vi "main.vi"() -> ()   [LabVIEW 2010]
uses:
  common_typedefs/channels_cluster.ctl
  common_typedefs/gate_parameters_cluster.ctl
  FPGAsubVIs/OnBoardBuffer/OnBoardBuffer.ctl
  FPGAsubVIs/write-to-fifo_status.ctl
  <vilib>/Platform/TimedLoop/XDataNode/XDataNode.xnode
  <vilib>/Platform/TimedLoop/XDataNode/timing_clust.ctl
  <vilib>/Platform/TimedLoop/XDataNode/nitl_modes.ctl
  <vilib>/Platform/TimedLoop/XDataNode/wakeup.ctl
  <vilib>/rvi/DataTransferAndStorage/Container/XNode/niFpgaContainer.xnode
  <vilib>/rvi/FIFO/Fifo_Resource/nirvififoEmulationSetSize.vi
  <vilib>/rvi/DataTransferAndStorage/Container/Common/niFpgaContainerGetUniqueNameForEmu.vi
  <vilib>/Platform/TimedLoop/XDataNode/XDNodeRunTimeDep.lvlib
  FPGAsubVIs/OnBoardBuffer/OnBoardBuffer.lvlib
panel:
  in  "clamp first pixel?":bool
  out "data received for buffering":u64
  out "local transfer FIFO full?":bool
  out "start acquisition?":bool
  out "write-to-FIFO status":T1
  out "on-board buffer":T2
  out "target-to-host FIFO full?":bool
  out "no. elements in on-board buffer":u32
  out "loop indicator":i32
  in  "gate 3":T3
  in  "gate 2":T3
  in  "gate 1":T3
  out "integrated pixel values":T4
  out "data read":T4
  in  "channel offsets":T4
  out "clock 3 state":bool
  out "clock 2 state":bool
  out "clock 1 state":bool
  in  "wait for trigger?":bool
  in  "stop":bool
  in  "acquire":bool
  out "acquiring?":bool
  out "current pixel no.":i64
  in  "number of pixels":i64=-1
  in  "maximum bit depth":i8
  in  "iterations per pixel":u32
  # "Outputs / displays"
  # "Integration parameters"
  # "Clock parameters"
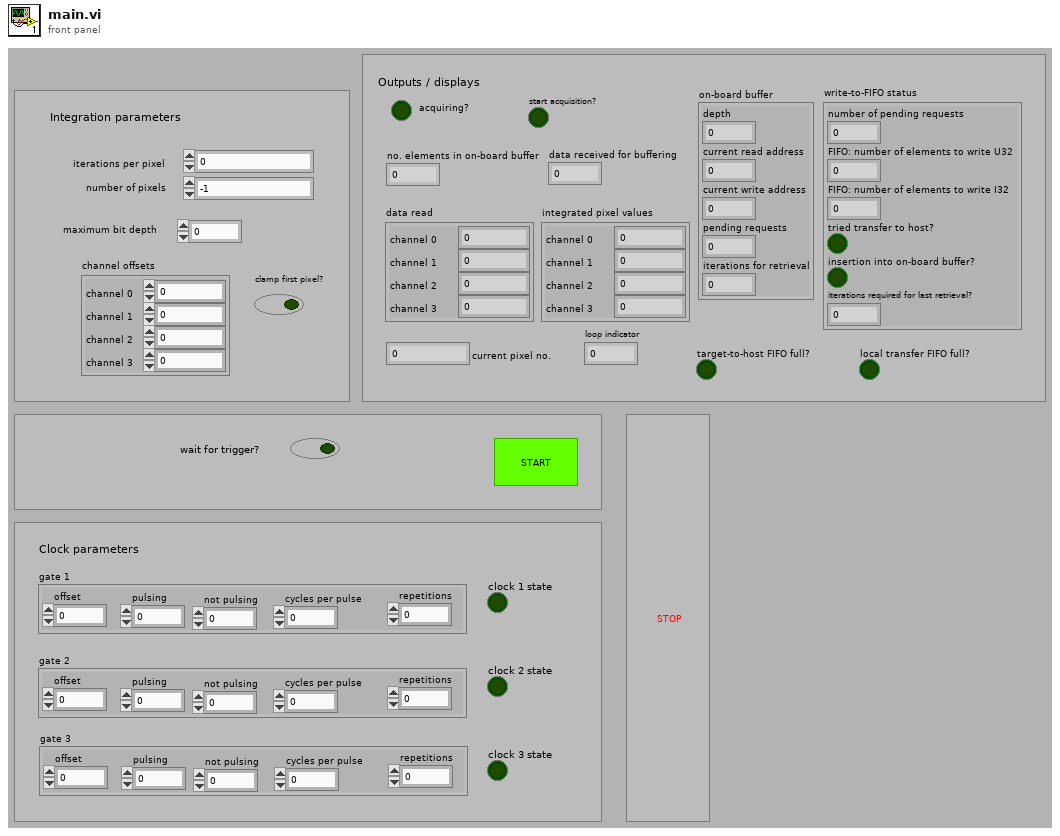
[diagram p1: front panel]
types:
  T1 = typedef "write-to-fifo_status.ctl" = cluster{"number of pending requests":i32, "FIFO: number of elements to write U32":u32, "FIFO: number of elements to write I32":i32, "tried transfer to host?":bool, "insertion into on-board buffer?":bool, "iterations required for last retrieval?":u32}
  T2 = typedef "OnBoardBuffer.lvlib/OnBoardBuffer.ctl" = cluster{"depth":u32, "current read address":u32, "current write address":u32, "pending requests":u32, "iterations for retrieval":u32}
  T3 = typedef "gate_parameters_cluster.ctl" = cluster{"offset":i64, "pulsing":i64, "not pulsing":i64, "cycles per pulse":i64, "repetitions":i64}
  T4 = typedef "channels_cluster.ctl" = cluster{"channel 0":u32, "channel 1":u32, "channel 2":u32, "channel 3":u32}
  T5 = typedef "XDNodeRunTimeDep.lvlib/timing_clust.ctl" = cluster{"Expected End [f-1]":u64, "Actual End [f-1]":u64, "Finished Late? [f-1]":bool, "Expected End [i-1]":u64, "Actual End [i-1]":u64, "Finished Late? [i-1]":bool, "Expected Start [i]":u64, "Actual Start [i]":u64, "Expected Start [f]":u64, "Actual Start [f]":u64, "Source Name":string, "Structure Name":string, "Period":i64, "Deadline":i64, "Offset":i64, "Start":i64, "Priority":i32, "Timeout":i32, "Mode":T6, "Wakeup Reason":T7, "Error":errorcluster, "Source Type":string, "Secondary Source Type":string, "Global End Time":u64, "Global Start Time":u64, "Frame Duration":u64, "Iteration Duration":u64, "Assigned CPU":i32, "I/O Scan Engine Mode":u32}
  T6 = typedef "XDNodeRunTimeDep.lvlib/nitl_modes.ctl" = enum32{"No Change", "Process missed periods, maintain original phase", "Discard missed periods, maintain original phase", "Process missed periods, ignore original phase", "Discard missed periods, ignore original phase"}
  T7 = typedef "XDNodeRunTimeDep.lvlib/wakeup.ctl" = enum32{"Normal", "Aborted", "Asynchronous wakeup", "Timing source error", "Timed loop error", "Timeout"}
  T8 = typedef "gate_counters_cluster.ctl" = cluster{"phase iteration counter":i64, "phase repetition counter":i64, "pulse iteration counter":i64, "phase state":bool}
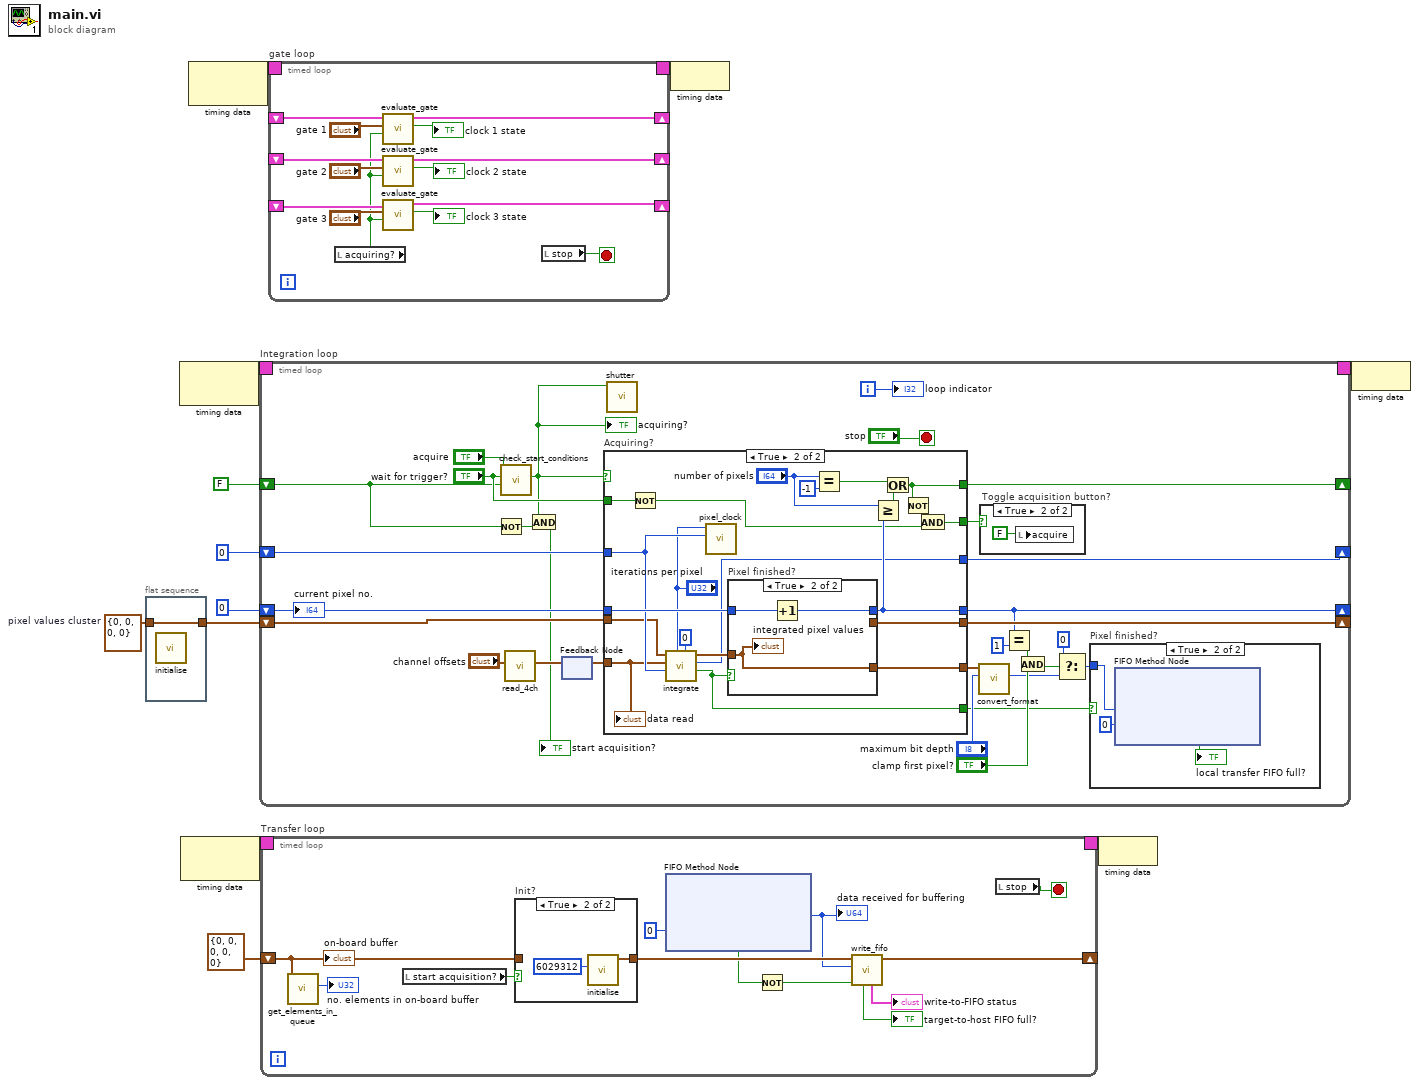
[diagram p0: block diagram]
diagram:
  w5 = T4 {"channel 0"=0, "channel 1"=0, "channel 2"=0, "channel 3"=0}  # pixel values cluster
  n1 = flat-sequence {
    tunnel: w5 -> [w13]
    tunnel: [w13] -> w4
    frame #0 {
      n2 = call "initialise.vi"() -> ()  [unwired: 12 in]
    }
  }
  n3 = node-c288() -> (w12:T5)  [unwired: 1 in]
  n4 = node-c288() -> (w2:T5)  [unwired: 1 in]
  n5 = node-c288() -> (w8:T5)  [unwired: 1 in]
  n6 = timed-loop "Integration loop" {
    timing: w12 -> [_]
    timing-out: [_] -> w11
    shift-right: [w19] -> _
    shift-left: i64 0 -> [w32]
    shift-right: [w37] -> _
    shift-left: u32 0 ("iteration counter out") -> [w39]
    shift-right: [w38] -> _
    shift-left: w4 -> [w40]
    shift-right: [w33] -> _
    shift-left: FALSE -> [w28]
    i -> [w29]
    stop <- "stop" stop-if-true
    n7 = Not(x=w28) -> (.not. x?=w26:bool)
    n8 = call "check_start_conditions.vi"("already acquiring?"=w28, "in triggered mode?"="wait for trigger?", "acquire"="acquire") -> ("acquire?"=w27:bool)  [unwired: 8 in]
    "acquiring?" <- w27
    n9 = call "read_4ch.vi"("channel offsets"="channel offsets") -> ("read output"=w35:T4)  [unwired: 10 in]
    n10 = And(x=w27, y=w26) -> (x .and. y?=→"start acquisition?":bool)
    n11 = feedback-in #1(w35) -> ()
    n12 = feedback #1() -> (w34:T4)  [unwired: 1 in]
    n13 = case "Acquiring?" shown="True" w27 {
      tunnel: [_ w105] -> w24
      tunnel: [_ w111] -> w37
      tunnel: [_ w115] -> w19
      tunnel: w40 -> [_ w108]
      tunnel: w32 -> [_ w113]
      tunnel: w39 -> [_ w110]
      tunnel: [_ w114] -> w38
      tunnel: w34 -> [_ w109]
      tunnel: [_ w103] -> w33
      tunnel: [_ w100] -> w30
      tunnel: "wait for trigger?" -> [_ w102]
      tunnel: [_ w98] -> w21
      frame False {
      }
      frame True {
        n14 = Not(x=w102) -> (.not. x?=w99:bool)
        n15 = call "integrate.vi"("waiting iterations per pixel"=u32 0, "integration iterations per pixel"="iterations per pixel", "iteration counter in"=w110, "sampling values in"=w109, "previous pixel values in"=w108) -> ("finished?"=w98:bool, "iteration counter out"=w111:u32, "new pixel values out"=w112:T4)  [unwired: 4 in]
        n16 = call "pixel_clock.vi"("current iteration"=w110, "iterations per pixel"="iterations per pixel") -> ()  [unwired: 10 in]
        n17 = case "Pixel finished?" shown="True" w98 {
          tunnel: w112 -> [w120 w123]
          tunnel: [_ w123] -> w105
          tunnel: [w119 w121] -> w115
          tunnel: w113 -> [w119 w122]
          tunnel: [w120 _] -> w114
          frame False {
          }
          frame True {
            n18 = Increment(x=w122) -> (x+1=w121:i64)
            "integrated pixel values" <- w123
          }
        }
        n19 = Equal?(x="number of pixels", y=i64 -1 ("x")) -> (x = y?=w118:bool)
        n20 = Greater Or Equal?(x="number of pixels", y=w115) -> (x >= y?=w117:bool)
        n21 = Or(x=w118, y=w117) -> (x .or. y?=w103:bool)
        n22 = Not(x=w103) -> (.not. x?=w101:bool)
        n23 = And(x=w101, y=w99) -> (x .and. y?=w100:bool)
        "data read" <- w109
      }
    }
    n24 = call "shutter.vi"("open?"=w27) -> ()  [unwired: 11 in]
    n25 = call "convert_format.vi"("maximum bit depth"="maximum bit depth", "values to be written"=w24) -> ("data"=w16:u64)  [unwired: 9 in]
    n26 = case "Toggle acquisition button?" shown="True" w30 {
      frame False {
      }
      frame True {
        n27 = local write "acquire"(FALSE) -> ()
      }
    }
    n28 = Equal?(x=w19, y=i64 1) -> (x = y?=w17:bool)
    n29 = And(x=w17, y="clamp first pixel?") -> (x .and. y?=w20:bool)
    n30 = Select(t=u64 0, s=w20, f=w16) -> (s? t:f=w15:u64)
    n31 = case "Pixel finished?" shown="True" w21 {
      tunnel: w15 -> [_ w45]
      frame False {
      }
      frame True {
        n32 = xnode ("FIFO Method Node")("Element"=w45, "Timeout"=0) -> ("Timed Out?"=→"local transfer FIFO full?":bool)  [unwired: 1 in, 1 out]
      }
    }
    "current pixel no." <- w32
    "loop indicator" <- w29
  }
  n33 = timed-loop "Transfer loop" {
    shift-right: [w133] -> _
    shift-left: T2 {"depth"=0, "current read address"=0, "current write address"=0, "pending requests"=0, "iterations for retrieval"=0} ("on-board buffer out") -> [w136]
    timing: w2 -> [_]
    timing-out: [_] -> w1
    stop <- w131 stop-if-true
    n34 = call "get_elements_in_queue.vi"("on-board buffer in"=w136) -> ("no. elements"=→"no. elements in on-board buffer":u32)  [unwired: 10 in]
    n35 = local read "start acquisition?"() -> (w135:bool)
    n36 = case "Init?" shown="True" w135 {
      tunnel: [w189 w191] -> w134
      tunnel: w136 -> [w189 _]
      frame False {
      }
      frame True {
        n37 = call "initialise.vi"("depth"=u32 6029312) -> ("on-board buffer out"=w191:T2)  [unwired: 10 in]
      }
    }
    n38 = xnode ("FIFO Method Node")("Timeout"=0) -> ("Element"=w130:u64, "Timed Out?"=w127:bool)  [unwired: 1 in, 1 out]
    "data received for buffering" <- w130
    n39 = Not(x=w127) -> (.not. x?=w126:bool)
    n40 = call "write_fifo.vi"("input ready?"=w126, "data"=w130, "on-board buffer in"=w134) -> ("on-board buffer out"=w133:T2, "write-to-FIFO status"=→"write-to-FIFO status":T1, "FIFO full?"=→"target-to-host FIFO full?":bool)  [unwired: 6 in]
    n41 = local read "stop"() -> (w131:bool)
    "on-board buffer" <- w136
  }
  n42 = timed-loop "gate loop" {
    timing: w8 -> [_]
    timing-out: [_] -> w7
    shift-right: [w206] -> _
    shift-left: _ -> [w207]
    shift-right: [w204] -> _
    shift-left: _ -> [w205]
    shift-right: [w203] -> _
    shift-left: _ -> [w202]
    stop <- w197 stop-if-true
    n43 = local read "acquiring?"() -> (w198:bool)
    n44 = call "evaluate_gate.vi"("acquiring?"=w198, "gate settings"="gate 1", "gate counters in"=w207) -> ("pulse state out"=→"clock 1 state":bool, "gate counters out"=w206:T8)  [unwired: 7 in]
    n45 = call "evaluate_gate.vi"("acquiring?"=w198, "gate settings"="gate 2", "gate counters in"=w205) -> ("pulse state out"=→"clock 2 state":bool, "gate counters out"=w204:T8)  [unwired: 7 in]
    n46 = call "evaluate_gate.vi"("acquiring?"=w198, "gate settings"="gate 3", "gate counters in"=w202) -> ("pulse state out"=→"clock 3 state":bool, "gate counters out"=w203:T8)  [unwired: 7 in]
    n47 = local read "stop"() -> (w197:bool)
  }
  n48 = node-c288(w7) -> ()
  n49 = node-c288(w1) -> ()
  n50 = node-c288(w11) -> ()
